vi "Read Scannable.vi"(8 "error in (no error)":errorcluster, 11 "Scanner.lvclass in":refnum<class "Scanner.lvclass">) -> (0 "error out":errorcluster, 2 "Scannable.lvclass":refnum<class "Scannable.lvclass">, 3 "Scanner.lvclass out":refnum<class "Scanner.lvclass">)   [LabVIEW 2017, in "Scanner.lvclass"]
doc: "(Protected) Return the Scannable object associated with this Scanner instance, to allow direct manipulation of that Instrument. Scannables are stored within Scanners, because LabVIEW does not allow inner classes. If inner classes were possible, it would be better to define Scanner as an inner class of Scannable."
uses:
  Scanner.lvclass
  Instruments/Utility Classes/Scannable/Scannable.lvclass
  Scanner.lvclass/Scanner.ctl
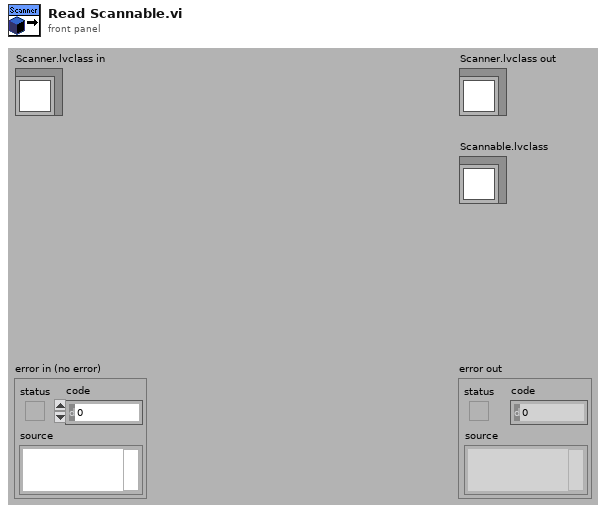
[diagram p1: front panel]
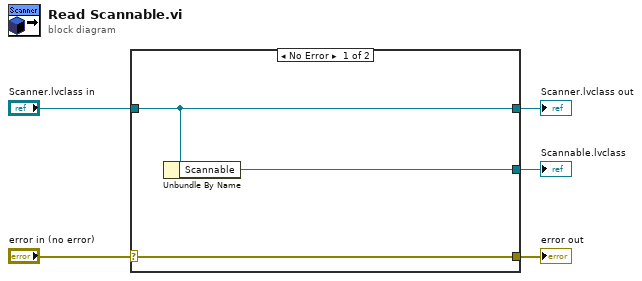
[diagram p0: block diagram]
diagram:
  n1 = case shown="No Error" "error in (no error)" {
    selector: "error in (no error)" -> [w8 w9]
    tunnel: [w8 w9] -> w4
    tunnel: [w7 w10] -> w2
    tunnel: "Scanner.lvclass in" -> [w7 w10]
    tunnel: [w6 _] -> w1
    frame No Error {
      n2 = Unbundle By Name(w7) -> ("Scannable"=w6:refnum<class "Scannable.lvclass">)
    }
    frame Error {
    }
  }
  "error out" <- w4
  "Scanner.lvclass out" <- w2
  "Scannable.lvclass" <- w1
